vi "ROI group-Extract selected groups data-Coore.vi"(11 "Indexes of ROI in group":i32[](array[numeric])) -> (0 "error IO":errorcluster, 1 "Points per cycle":u16, 3 "ROI group data":T1)   [LabVIEW 2017]
uses:
  xcontrol/Interface VIs/Interface typedefs/Interface-Data format definition.ctl
  xcontrol/Typedefs/Xctl-XY data type definition.ctl
  xcontrol/Typedefs/Xctrl-ROI type enum.ctl
  xcontrol/Interface VIs/Interface typedefs/Interface-Data array.ctl
  Experiment header interface/Typedefs/Header parameters cluster-Zstack.ctl
  Typedefs/Frame Size.ctl
  Global variables/gl_Functional Imaging-Global variables.vi
  xcontrol/XGrapher.xctl
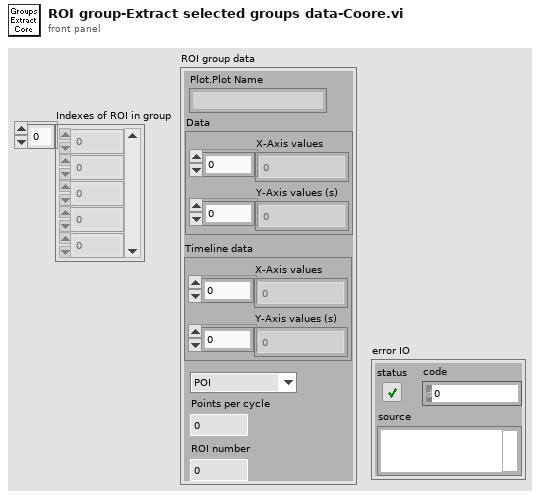
[diagram p1: front panel]
types:
  T1 = typedef "Interface-Data format definition.ctl" = cluster{"Plot.Plot Name":string, "Data":T2, "Timeline data":T2, "Type":T3, "Points per cycle":u16, "ROI number":u16}
  T2 = typedef "XGrapher.xctl/Xctl-XY data type definition.ctl" = cluster{"X-Axis values":sgl[], "Y-Axis values (s)":sgl[]}
  T3 = typedef "Xctrl-ROI type enum.ctl" = enum16{"POI", "Mini-scan", "Group"}
  T4 = typedef "Header parameters cluster-Zstack.ctl" = cluster{"Number of POI":u16, "Number of Miniscans":u16, "Number of Trials":u16, "Number of Cycles ":u16, "# Averaged Frames":u16, "Laser power (%)":u8, "Pockels":dbl, "Acquisition Length (sec)":dbl, "Fill time (us)":dbl, "DwellTime (us)":dbl, "Miniscan Dwell time per pixel (us)":dbl, "PMT 1":dbl, "PMT 2":dbl, "Back Apperture":dbl, "Zoom":dbl, "Number of Pixels in Miniscan":u16, "Frame Size":T5, "Field of View":dbl, "X centre":dbl, "Y centre":dbl, "AOL Z":dbl}
  T5 = typedef "Frame Size.ctl" = u16
  T6 = cluster{"Channel A?":bool, "Cycle length (us)":dbl, "[Pixels in ROI]":i32[], "Z-Stack Header data":T4, "[ROI Time (us)]":dbl[], "Path out":path, "Version index":i32}
  T7 = typedef "Interface-Data array.ctl" = T1[]
  T8 = typedef "Functional Imging UI Refs.ctl" = cluster{"Menu ref":refnum<k9>, "Image control":refnum<vi>, "VI ref":refnum<vi>, "XGrapher":refnum<vi>, "Smoothing":refnum<vi>, "POI Averaging":refnum<vi>, "Normalize":refnum<vi>, "POI data points in each trial":refnum<vi>, "Channel":refnum<vi>, "Experiment data folder path":refnum<vi>, "[ROI vis]":refnum<vi>, "[Groups] visbl":T9, "Group Name":refnum<vi>, "POI index":refnum<vi>, "Trial No.":refnum<vi>, "Intensity Zoom":refnum<vi>, "Trial Cursor Enabled":refnum<vi>, "Number of Trials (ind 1)":refnum<vi>, "Number of Trials (ind 2)":refnum<vi>, "MiniScans Available":refnum<vi>, "POI Available":refnum<vi>, "Defer graph updates":refnum<vi>, "Waveform selector":refnum<vi>, "#of selected POI":refnum<vi>, "#of selected MiniScans":refnum<vi>, "#of selected groups":refnum<vi>, "Max Z-Projection":refnum<vi>, "Z-Plane Selector":refnum<vi>, "Index of miniscan point to visualise":refnum<vi>, "ROI vis. mode":refnum<vi>, "Total # of points":refnum<vi>, "Index of group clicked on":refnum<vi>, "Pane 1":refnum<vi>, "Pane 2":refnum<vi>, "Pane 3":refnum<vi>, "Pane 4":refnum<vi>, "Pane 5":refnum<vi>, "Pane 6":refnum<vi>, "Deselect all ROI":refnum<vi>, "Deselect all groups":refnum<vi>}
  T9 = typedef "Groups array referecne.ctl" = refnum<vi>
  T10 = typedef "ROI selector array-ROI vis.ctl" = T11[]
  T11 = typedef "Interface-ROI selection cluster.ctl" = cluster{"ROI number":i32, "ROI ID":T12, "Visibility":bool}
  T12 = typedef "ROI ID Enum.ctl" = enum16{"Point", "MiniScan", "Comp. MiniScan", "Rectangle", "Comp. volume", "Arb. plane point", "None"}
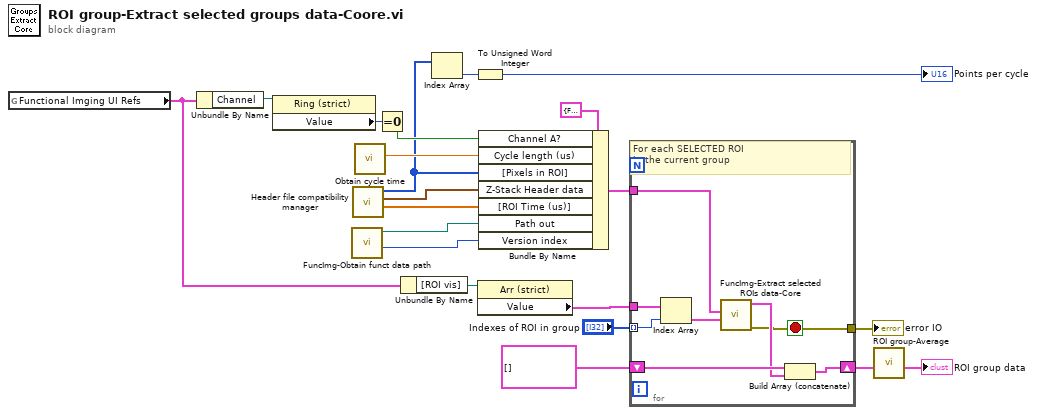
[diagram p0: block diagram]
diagram:
  n1 = global read "gl_Functional Imaging-Global variables.vi" "Functional Imging UI Refs"() -> (w13:T8)
  n2 = Unbundle By Name(w13) -> ("Channel"=w10:refnum<vi>)
  n3 = property on="Property Node" class="Ring (strict)"(reference=w10) -> ("Value"=w20:u16)  [unwired: 1 in, 2 out]
  n4 = call "FuncImg-Obtain funct data path.vi"() -> ("Version index (-1 = latest version)"=w19:i32, "Functional data folder path"=w18:path)  [unwired: 7 in, 3 out]
  n5 = call "Header file compatibility manager.vi"() -> ("[ROI Time (us)]"=w17:dbl[], "Z-Stack Header data"=w16:T4, "[Pixels in ROI]"=w7:i32[])  [unwired: 8 in, 1 out]
  n6 = call "Obtain cycle time.vi"() -> ("Funct Acq cycle length (us)"=w14:dbl)  [unwired: 9 in, 2 out]
  n7 = Equal To 0?(x=w20) -> (x = 0?=w21:bool)
  n8 = Unbundle By Name(w13) -> ("[ROI vis]"=w11:refnum<vi>)
  n9 = Index Array(array=w7) -> (element=w6:i32)  [unwired: 1 in]
  n10 = To Unsigned Word Integer(number=w6) -> (unsigned 16bit integer=→"Points per cycle":u16)
  n11 = property on="Property Node" class="Arr (strict)"(reference=w11) -> ("Value"=w9:T10)  [unwired: 1 in, 2 out]
  n12 = Bundle By Name(cluster=T6 {"Channel A?"=FALSE, "Cycle length (us)"=0.0, "[Pixels in ROI]"=[], "Z-Stack Header data"={"Number of POI"=0, "Number of Miniscans"=0, "Number of Trials"=0, "Number of Cycles "=0, "# Averaged Frames"=0, "Laser power (%)"=0, "Pockels"=0.0, "Acquisition Length (sec)"=0.0, "Fill time (us)"=0.0, "DwellTime (us)"=0.0, "Miniscan Dwell time per pixel (us)"=0.0, "PMT 1"=0.0, "PMT 2"=0.0, "Back Apperture"=0.0, "Zoom"=0.0, "Number of Pixels in Miniscan"=0, "Frame Size"=200, "Field of View"=0.0, "X centre"=0.0, "Y centre"=0.0, "AOL Z"=0.0}, "[ROI Time (us)]"=[], "Path out"=path "", "Version index"=0} ("Cluster"), "Channel A?"=w21, "Cycle length (us)"=w14, "[Pixels in ROI]"=w7, "Z-Stack Header data"=w16, "[ROI Time (us)]"=w17, "Path out"=w18, "Version index"=w19) -> (w15:T6)
  n13 = for {
    tunnel: w9 -> [w27]
    shift-right: [w29] -> w4
    shift-left: T7 [] ("element") -> [w28]
    tunnel: "Indexes of ROI in group" -> [w25] mode=indexing
    tunnel: w15 -> [w24]
    tunnel: [w22] -> w2
    stop <- w22 stop-if-true
    # "For each SELECTED ROI\nin the current group"
    n14 = Index Array(array=w27, index=w25) -> (element=w26:T11)
    n15 = call "FuncImg-Extract selected ROIs data-Core.vi"("System Cluster"=w26, "Input cluster"=w24) -> ("error IO"=w22:errorcluster, "Interface-Data format definition"=w23:T1)  [unwired: 7 in, 1 out]
    n16 = Build Array (concatenate)(w28, w23) -> (w29:T7)
  }
  "error IO" <- w2
  n17 = call "ROI group-Average.vi"("Data in"=w4) -> ("ROI group data"=→"ROI group data":T1)  [unwired: 9 in, 1 out]
